vi "Hash Type to Int.vi"(1 "Type":T1) -> (0 "i32":i32)   [LabVIEW 2017, in "Toolkit.lvlib" / "Session.lvclass"]
uses:
  Session.lvclass
  API/Typedefs/Host Key Hash Types.ctl
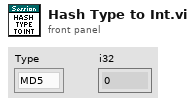
[diagram p1: front panel]
types:
  T1 = typedef "Toolkit.lvlib/Session.lvclass/Host Key Hash Types.ctl" = enum32{"MD5", "SHA1"}
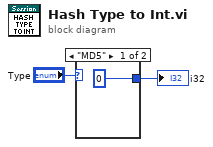
[diagram p0: block diagram]
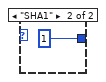
[diagram p2: hidden frame]
diagram:
  n1 = case shown="\"MD5\"" "Type" {
    tunnel: [0 1] -> w2
    frame "MD5" {
    }
    frame "SHA1" {
    }
  }
  "i32" <- w2
